vi "Parse Packet Header.vi"(8 "error in (no error)":errorcluster, 10 "Bytes in":u8[](array[numeric]), 11 "pcap Parse and Build in":refnum<class "pcap Parse and Build.lvclass">) -> (0 "error out":errorcluster, 1 "Packet Header":T1, 2 "Bytes out":u8[](array[numeric]), 3 "pcap Parse and Build out":refnum<class "pcap Parse and Build.lvclass">, 4 "TAI Time (ns)":i64, 5 "Next Packet offset":i32)   [LabVIEW 2021, in "pcap Parse and Build.lvclass"]
uses:
  pcap Parse and Build.lvclass
  pcap Parse and Build.lvclass/pcap Parse and Build.ctl
  Typedef/Packet Header.ctl
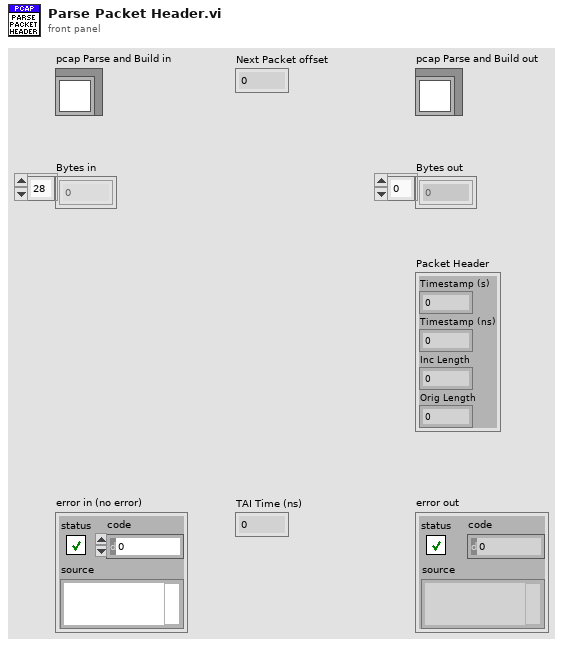
[diagram p1: front panel]
types:
  T1 = typedef "pcap Parse and Build.lvclass/Packet Header.ctl" = cluster{"Timestamp (s)":u32, "Timestamp (ns)":u32, "Inc Length":u32, "Orig Length":u32}
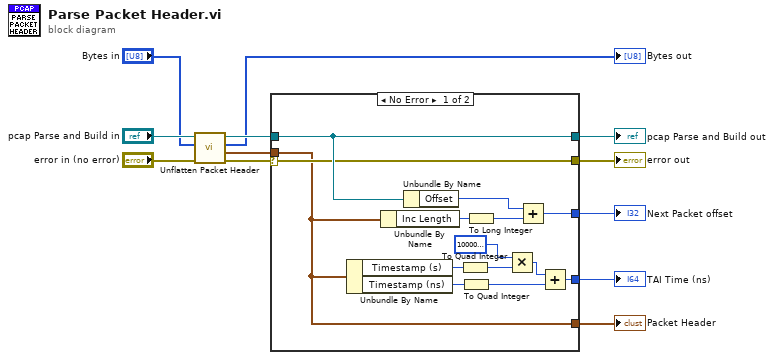
[diagram p0: block diagram]
diagram:
  n1 = call "Unflatten Packet Header.vi"("error in (no error)"="error in (no error)", "Bytes in"="Bytes in", "pcap Parse and Build in"="pcap Parse and Build in") -> ("error out"=w2:errorcluster, "Packet Header"=w1:T1, "Bytes out"=→"Bytes out":u8[], "pcap Parse and Build out"=w6:refnum<class "pcap Parse and Build.lvclass">)  [unwired: 5 in]
  n2 = case shown="No Error" w2 {
    selector: w2 -> [w14 w28]
    tunnel: [w14 w28] -> w9
    tunnel: [w13 _] -> w12
    tunnel: [w20 _] -> w11
    tunnel: [w17 _] -> w10
    tunnel: w6 -> [w15 w27]
    tunnel: [w15 w27] -> w8
    tunnel: w1 -> [w13 _]
    frame No Error {
      n3 = Unbundle By Name(w13) -> ("Timestamp (s)"=w26:u32, "Timestamp (ns)"=w25:u32)
      n4 = Unbundle By Name(w13) -> ("Inc Length"=w19:u32)
      n5 = Unbundle By Name(w15) -> ("Offset"=w16:i32)
      n6 = To Quad Integer(1:w26) -> (0:w24:i64)
      n7 = To Quad Integer(1:w25) -> (0:w22:i64)
      n8 = To Long Integer(number=w19) -> (32bit integer=w18:i32)
      n9 = Multiply(x=i64 1000000000, y=w24) -> (x*y=w21:i64)
      n10 = Add(x=w16, y=w18) -> (x+y=w17:i32)
      n11 = Add(x=w21, y=w22) -> (x+y=w20:i64)
    }
    frame Error {
    }
  }
  "error out" <- w9
  "pcap Parse and Build out" <- w8
  "Packet Header" <- w12
  "TAI Time (ns)" <- w11
  "Next Packet offset" <- w10
